vi "Create and Add Instruments.vi"(6 "Physical Instr CFGs":string[](array[string]), 7 "Enqueuers":T1(c390), 8 "Error In":errorcluster, 11 "Target Measure and Stimulus Subsystems in":refnum<class "Target Measure and Stimulus Subsystems.lvclass">) -> (0 "Error Out":errorcluster, 3 "Target Measure and Stimulus Subsystems out":refnum<class "Target Measure and Stimulus Subsystems.lvclass">)   [LabVIEW 2023, in "HAL GOOP4.lvlib" / "Target Measure and Stimulus Subsystems.lvclass"]
uses:
  Target Measure and Stimulus Subsystems.lvclass
  Target Measure and Stimulus Subsystems.lvclass/Target Measure and Stimulus Subsystems.ctl
  <vilib>/Utility/error.llb/Error Cluster From Error Code.vi
  <vilib>/ErrorRing/Error Ring.xnode
  bed49599-bcdd-41cd-8160-b042be87718c.vi
  Configuration/Configuration JSON/Configuration JSON Base/CFG JSON.lvclass
  Instrument/Instrument.lvclass
  Host Measure and Stimulus Subsystems/Host Measure and Stimulus Subsystems.lvclass
  <vilib>/ActorFramework/Message Enqueuer/Message Enqueuer.lvclass
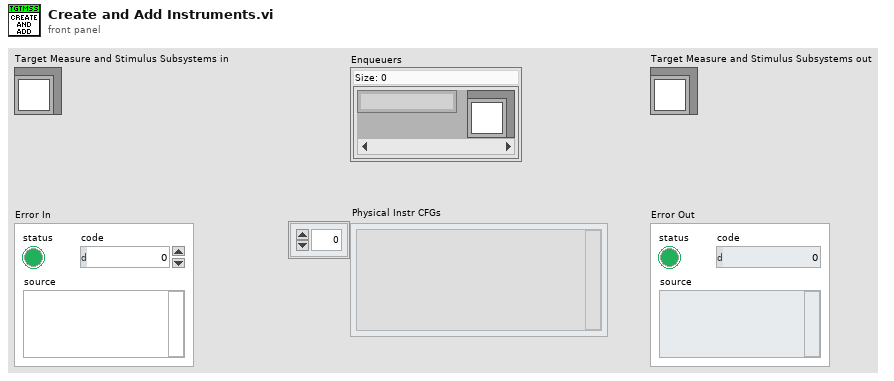
[diagram p1: front panel]
types:
  T1 = map{string, refnum<class "Message Enqueuer.lvclass">}
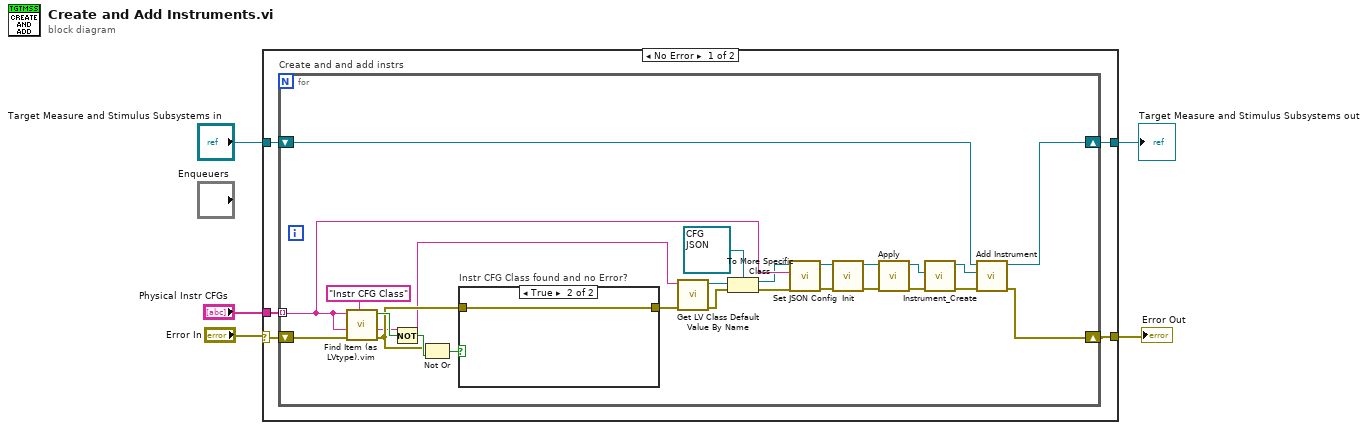
[diagram p0: block diagram]
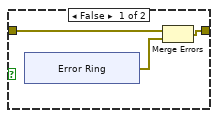
[diagram p2: hidden frame]
diagram:
  n1 = case shown="No Error" "Error In" {
    selector: "Error In" -> [w7 w45]
    tunnel: [w8 w45] -> w1
    tunnel: [w9 w46] -> w2
    tunnel: "Target Measure and Stimulus Subsystems in" -> [w10 w46]
    tunnel: "Physical Instr CFGs" -> [w6 _]
    frame No Error {
      n2 = for "Create and and add instrs" {
        shift-right: [w27] -> w8
        shift-left: w7 -> [w28]
        tunnel: w6 -> [w24] mode=indexing
        shift-right: [w25] -> w9
        shift-left: w10 -> [w26]
        n3 = call "Find Item (as LVtype).vim"("$Path or Item Name"="Instr CFG Class", "error in (no error)"=w28, "Data Type and Default Value"=w24, "JSON"=w24) -> ("error out"=w31:errorcluster, "Data"=w29:string, "Found"=w33:bool)  [unwired: 4 in, 1 out]
        n4 = Not(x=w33) -> (.not. x?=w35:bool)
        n5 = Not Or(1:w35, 2:w31) -> (0:w34:bool)
        n6 = case "Instr CFG Class found and no Error?" shown="True" w34 {
          tunnel: [w38 w44] -> w32
          tunnel: w31 -> [w36 w44]
          frame False {
            n7 = xnode "Error Ring"() -> ("error out"=w37:errorcluster)
            n8 = Merge Errors(w36, w37) -> (w38:errorcluster)
          }
          frame True {
          }
        }
        n9 = call <vilib>:"Get LV Class Default Value By Name.vi"("error in (no error)"=w32, "class name"=w29) -> ("error out"=w23:errorcluster, "object"=w22:refnum<class>)  [unwired: 8 in]
        n10 = To More Specific Class(target class=refnum<class "CFG JSON.lvclass"> refnum ("HAL GOOP4.lvlib:CFG JSON Base.lvclass"), reference=w22, error in=w23) -> (specific class reference=w18:refnum<class "CFG JSON.lvclass">, error out=w17:errorcluster)
        n11 = call "Set JSON Config.vi"("error in (no error)"=w17, "<JSON>Config>"=w24, "CFG Base in"=w18) -> ("error out"=w20:errorcluster, "CFG Base out"=w15:refnum<class "CFG JSON.lvclass">)  [unwired: 7 in]
        n12 = call-dynamic "Init.vi"("error in (no error)"=w20, "IConfigure in"=w15) -> ("error out"=w16:errorcluster, "IConfigure out"=w13:refnum<class "CFG JSON.lvclass">)  [unwired: 8 in]
        n13 = call-dynamic "Apply.vi"("error in (no error)"=w16, "IConfigure in"=w13) -> ("error out"=w14:errorcluster, "IConfigure out"=w12:refnum<class "CFG JSON.lvclass">)  [unwired: 8 in]
        n14 = call "Instrument_Create.vi"("Error In"=w14, "IConfigure"=w12) -> ("Error Out"=w21:errorcluster, "reference out"=w11:refnum<class "Instrument.lvclass">)  [unwired: 8 in]
        n15 = call "Add Instrument.vi"("error in"=w21, "Instrument"=w11, "Host Measure and Stimulus Subsystems in"=w26) -> ("error out"=w27:errorcluster, "Host Measure and Stimulus Subsystems out"=w25:refnum<class "Target Measure and Stimulus Subsystems.lvclass">)  [unwired: 7 in]
      }
    }
    frame Error {
    }
  }
  "Target Measure and Stimulus Subsystems out" <- w2
  "Error Out" <- w1
